vi "StopProcess.vi"(0 "reference in":refnum<class "VCS.lvclass">, 2 "ms timeout (-1)":i32=-1, 5 "Error In":errorcluster) -> (14 "reference out":refnum<class "VCS.lvclass">, 19 "Error Out":errorcluster)   [LabVIEW 2023, in "VCS.lvclass"]
uses:
  VCS.lvclass
  VCS.lvclass/VCS.ctl
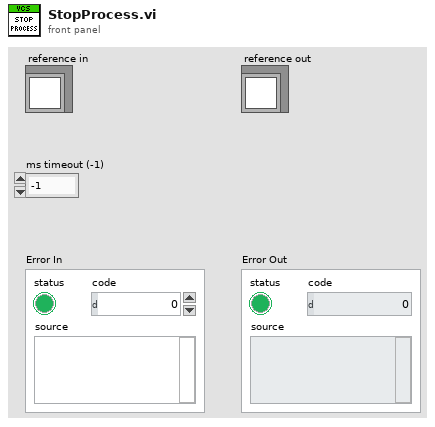
[diagram p1: front panel]
types:
  T1 = enum16{"ReadRepository", "CreateNew", "CreateOrLookUpExisting", "ReadRepositoryAndDestroy"}
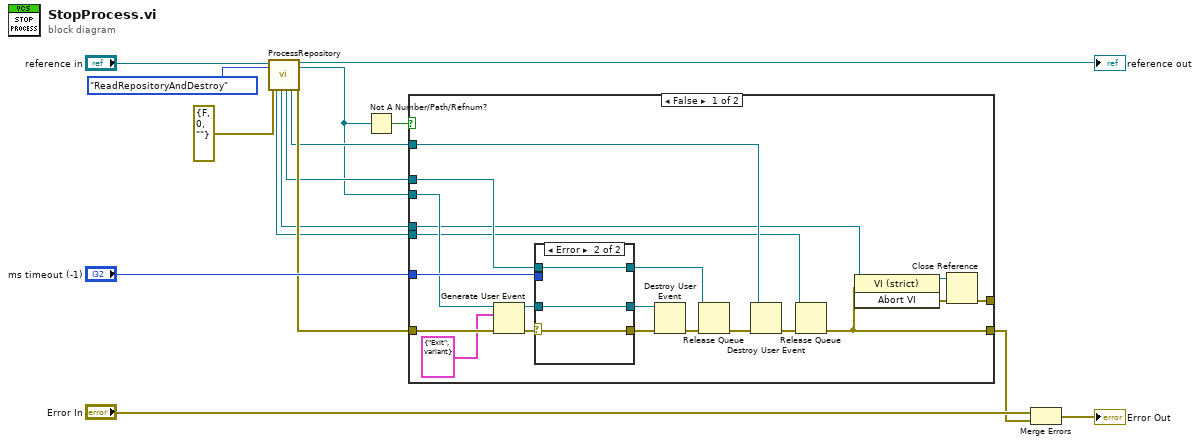
[diagram p0: block diagram]
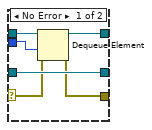
[diagram p2: hidden frame]
diagram:
  n1 = call "ProcessRepository.vi"("reference in"="reference in", "Action(ReadRepository)"=T1."ReadRepositoryAndDestroy", "Error In"=errorcluster {"status"=FALSE, "code"=0, "source"=""} ("error in (no error)")) -> ("QueueFromProcess"=w2:refnum<queue>, "ProcessViRef"=w6:refnum<vi>, "ProcessSyncQueue"=w8:refnum<queue>, "EventFromProcess"=w7:refnum<user-event>, "reference out"=→"reference out":refnum<class "VCS.lvclass">, "EventsToProcess"=w4:refnum<user-event>, "Error Out"=w9:errorcluster)  [unwired: 9 in, 1 out]
  n2 = Not A Number/Path/Refnum?(number/path/refnum=w4) -> (NaN/Path/Refnum?=w3:bool)
  n3 = case shown="False" w3 {
    tunnel: w8 -> [w35 _]
    tunnel: w9 -> [w28 w45]
    tunnel: [w16 w45] -> w13
    tunnel: w4 -> [w27 _]
    tunnel: "ms timeout (-1)" -> [w31 _]
    tunnel: w7 -> [w29 _]
    tunnel: w6 -> [w25 _]
    tunnel: w2 -> [w21 _]
    tunnel: [w17 _] -> _
    frame False {
      n4 = Generate User Event(user event=w27, event data cluster=cluster{"Command":string, "Data":variant} {"Command"="Exit", "Data"=variant} ("event data"), error in=w28) -> (user event out=w34:refnum<user-event>, error out=w30:errorcluster)  [unwired: 1 in]
      n5 = case shown="Error" w30 {
        tunnel: [w39 w44] -> w33
        tunnel: w35 -> [w38 w42]
        tunnel: [w41 w43] -> w32
        tunnel: w34 -> [w41 w43]
        tunnel: w31 -> [w37 _]
        selector: w30 -> [w40 w44]
        tunnel: [w36 w42] -> w18
        frame No Error {
          n6 = Dequeue Element(queue=w38, timeout in ms (-1)=w37, error in (no error)=w40) -> (queue out=w36:refnum<queue>, error out=w39:errorcluster)  [unwired: 2 out]
        }
        frame Error {
        }
      }
      n7 = Destroy User Event(user event=w32, error in=w33) -> (error out=w20:errorcluster)
      n8 = Release Queue(queue=w18, error in (no error)=w20) -> (error out=w19:errorcluster)  [unwired: 1 in, 2 out]
      n9 = Destroy User Event(user event=w29, error in=w19) -> (error out=w22:errorcluster)
      n10 = Release Queue(queue=w21, error in (no error)=w22) -> (error out=w16:errorcluster)  [unwired: 1 in, 2 out]
      n11 = invoke class="VI (strict)" method="Abort VI"(reference=w25, error in=w16) -> (reference out=w24:refnum<vi>, error out=w23:errorcluster)  [unwired: 1 in, 1 out]
      n12 = Close Reference(reference=w24, error in (no error)=w23) -> (error out=w17:errorcluster)
    }
    frame True {
    }
  }
  n13 = Merge Errors("Error In", w13) -> (→"Error Out":errorcluster)
